vi "Cleanup Log Folder.vi"(7 "Template":string, 8 "Error In":errorcluster, 9 "Min Fraction":dbl=0.2, 10 "Min Space":i64, 11 "Log File Path In":path) -> (0 "Error Out":errorcluster)   [LabVIEW 2021]
panel:
  out "Log File Path Out":path
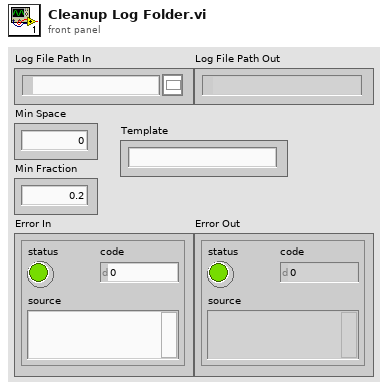
[diagram p1: front panel]
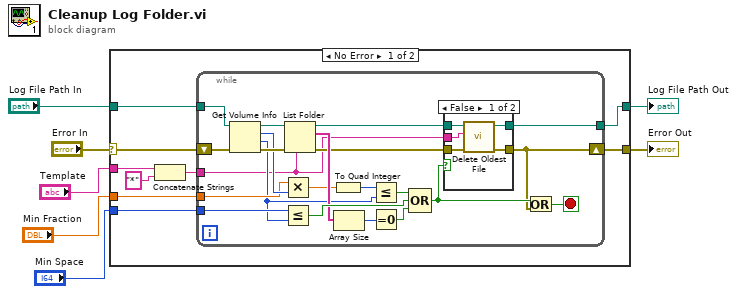
[diagram p0: block diagram]
diagram:
  n1 = case shown="No Error" "Error In" {
    selector: "Error In" -> [w8 w46]
    tunnel: "Min Space" -> [w16 _]
    tunnel: [w15 w46] -> w6
    tunnel: "Log File Path In" -> [w14 w47]
    tunnel: "Template" -> [w13 _]
    tunnel: "Min Fraction" -> [w10 _]
    tunnel: [w9 w47] -> w2
    frame No Error {
      n2 = Concatenate Strings(w13, "*" ("string")) -> (w12:string)
      n3 = while {
        shift-right: [w29] -> w15
        shift-left: w8 -> [w38]
        tunnel: w14 -> [w28]
        tunnel: w16 -> [w25]
        tunnel: w12 -> [w17]
        tunnel: w10 -> [w23]
        tunnel: [w18] -> w9
        stop <- w30 stop-if-true
        n4 = Get Volume Info(8:w38, 11:w28) -> (0:w37:errorcluster, 1:w20:i64, 2:w24:i64, 3:w27:path)  [unwired: 2 out]
        n5 = Multiply(x=w23, y=w24) -> (x*y=w22:dbl)
        n6 = Less Or Equal?(x=w25, y=w20) -> (x <= y?=w36:bool)
        n7 = List Folder(path=w27, pattern=w17, error in=w37) -> (path out=w26:path, filenames=w35:string[], error out=w31:errorcluster)  [unwired: 1 in, 1 out]
        n8 = To Quad Integer(1:w22) -> (0:w21:i64)
        n9 = Array Size(array=w35) -> (size(s)=w34:i32)
        n10 = Less Or Equal?(x=w21, y=w20) -> (x <= y?=w19:bool)
        n11 = Equal To 0?(x=w34) -> (x = 0?=w33:bool)
        n12 = Compound Arithmetic op=OR(w19, w36, w33) -> (w32:bool)
        n13 = case shown="False" w32 {
          tunnel: w31 -> [w42 w45]
          tunnel: w26 -> [w43 w44]
          tunnel: [w41 w45] -> w29
          tunnel: [w40 w44] -> w18
          tunnel: w17 -> [w39 _]
          frame False {
            n14 = call "Delete Oldest File.vi"("error in"=w42, "pattern"=w39, "path"=w43) -> ("error out"=w41:errorcluster, "path out"=w40:path)  [unwired: 7 in]
          }
          frame True {
          }
        }
        n15 = Or(x=w32, y=w29) -> (x .or. y?=w30:bool)
      }
    }
    frame Error {
    }
  }
  "Error Out" <- w6
  "Log File Path Out" <- w2
